vi "Display Options Window.vi"(8 "error in (no error)":errorcluster, 11 "Feed Module State Cluster in":T1={"Shared Variables"={"PID 1 Process Variable"="PID1-Mettler Toledo Scale 1", "PID 1 Output"="PID1-Mettler Toledo Scale 1", "PID 1 Setpoint"="PID1-Setpoint", "PID 1 Setpoint SV refnum"="ni.var.psp://localhost/Flow Module 1/PID1-Setpoint", "PID 1 Process Variable SV refnum"="ni.var.psp://localhost/Flow Module 1/PID1-Setpoint", "PID 1 Output SV refnum"="ni.var.psp://localhost/Flow Module 1/PID1-Setpoint"}, "Feed Module Config"={"GUID"="", "Drop Coords"={"Horizontal"=0, "Vertical"=0}, "Process Name"="", "User name"="", "Queue Name"="", "Settings"={"Cycle Period"=500.0, "Ismatech"={"VISA resource name"="", "Simulated?"=TRUE, "Pump Number"=1.0, "Reverse?"=FALSE}, "Masterflex"={"VISA resource name"="", "Simulated?"=TRUE, "Pump Number"=1.0, "Reverse?"=FALSE}, "Mettler"={"VISA resource name"="", "Simulated?"=FALSE}, "Bronkhorst M13 Flow Meter"={"VISA resource name"="", "Simulated?"=TRUE, "Smoothing Steps"=1}, "PID 2 Parameters"={"Input Device"=enum."Default", "Output Device"=enum."Default", "Setpoint"=0.0, "PID gains"={"proportional gain (Kc)"=1.0, "integral time (Ti, min)"=0.01, "derivative time (Td, min)"=0.0}}, "Manual Entry"=0.0, "Auto?"=TRUE, "PID range"={"PID High"=100.0, "PID Low"=0.0, "High Warning"=100.0}, "Tacmina Settings"={"Analog DAQ Task"="", "Digital DAQ Task"=""}, "KNF SIMDOS Settings"={"VISA resource name"="", "Simulated?"=TRUE}, "ASIA Pump C"={"ASIA Pump #"=0, "channel"=0, "Simulated"=FALSE}, "VICI Settings"={"VISA resource name"="", "Pump ID"="", "Pump Head Vol"=0.0, "Reverse?"=FALSE, "Simulated?"=TRUE}, "FLOM Settings"={"VISA resource name"="", "Simulated?"=TRUE, "Pump Number"=0.0}, "SSI PR/LD Settings"={"VISA resource name"="", "Simulated?"=FALSE}, "Masterflex 75211 Settings"={"Analog DAQ Task"="", "Digital DAQ Task"=""}, "SSI P40 Settings"={"VISA resource name"="", "Simulated?"=TRUE}, "Ismatech 3 Channel Settings"={"VISA resource name"="", "Pump Number"=1, "Channel Number"=0, "Simulated?"=TRUE, "Reverse?"=FALSE}, "Bronkhorst M14 Settings"={"VISA resource name"="", "Simulated?"=FALSE, "Smoothing Steps"=1}, "Reset Totalizer"=FALSE, "Input Num Alarm Settings"=[], "Control Type"=enum."g/min", "Front End Display Options"={"Temperature"=TRUE, "Scale Grams"=FALSE, "Density"=TRUE, "Flow (g/min)"=FALSE, "Flow (ml/min)"=TRUE, "PSIG"=TRUE, "Total Grams"=TRUE, "Updated"=TRUE}}, "Settings Load Count"=0, "OP Load Count"=0}} {"Feed Module Config"."Settings"."Bronkhorst M14 Settings"."Smoothing Steps" min=1 step=1; "Feed Module Config"."Settings"."Ismatech 3 Channel Settings"."Channel Number" min=0 max=3; "Feed Module Config"."Settings"."Ismatech 3 Channel Settings"."Pump Number" min=1; "Feed Module Config"."Settings"."PID range"."PID Low" min=0.0 max=100.0 format="%.2f"; "Feed Module Config"."Settings"."PID range"."PID High" format="%.2f"; "Feed Module Config"."Settings"."PID 2 Parameters"."PID gains"."derivative time (Td, min)" format="%.3f"; "Feed Module Config"."Settings"."PID 2 Parameters"."PID gains"."integral time (Ti, min)" format="%.3f"; "Feed Module Config"."Settings"."PID 2 Parameters"."PID gains"."proportional gain (Kc)" format="%.3f"; "Feed Module Config"."Settings"."Bronkhorst M13 Flow Meter"."Smoothing Steps" min=1 step=1; "Feed Module Config"."Settings"."ASIA Pump C"."channel" min=0 max=1 step=1; "Feed Module Config"."Settings"."Ismatech"."Pump Number" min=1.0 max=20.0 step=1.0; "Feed Module Config"."Settings"."Masterflex"."Pump Number" min=1.0 max=20.0 step=1.0}) -> (0 "error out":errorcluster, 2 "Updated in DO":bool, 3 "Feed Module State Cluster out":T1={"Shared Variables"={"PID 1 Process Variable"="PID1-Mettler Toledo Scale 1", "PID 1 Output"="PID1-Mettler Toledo Scale 1", "PID 1 Setpoint"="PID1-Setpoint", "PID 1 Setpoint SV refnum"="ni.var.psp://localhost/Flow Module 1/PID1-Setpoint", "PID 1 Process Variable SV refnum"="ni.var.psp://localhost/Flow Module 1/PID1-Setpoint", "PID 1 Output SV refnum"="ni.var.psp://localhost/Flow Module 1/PID1-Setpoint"}, "Feed Module Config"={"GUID"="", "Drop Coords"={"Horizontal"=0, "Vertical"=0}, "Process Name"="", "User name"="", "Queue Name"="", "Settings"={"Cycle Period"=500.0, "Ismatech"={"VISA resource name"="", "Simulated?"=TRUE, "Pump Number"=1.0, "Reverse?"=FALSE}, "Masterflex"={"VISA resource name"="", "Simulated?"=TRUE, "Pump Number"=1.0, "Reverse?"=FALSE}, "Mettler"={"VISA resource name"="", "Simulated?"=FALSE}, "Bronkhorst M13 Flow Meter"={"VISA resource name"="", "Simulated?"=TRUE, "Smoothing Steps"=1}, "PID 2 Parameters"={"Input Device"=enum."Default", "Output Device"=enum."Default", "Setpoint"=0.0, "PID gains"={"proportional gain (Kc)"=1.0, "integral time (Ti, min)"=0.01, "derivative time (Td, min)"=0.0}}, "Manual Entry"=0.0, "Auto?"=TRUE, "PID range"={"PID High"=100.0, "PID Low"=0.0, "High Warning"=100.0}, "Tacmina Settings"={"Analog DAQ Task"="", "Digital DAQ Task"=""}, "KNF SIMDOS Settings"={"VISA resource name"="", "Simulated?"=TRUE}, "ASIA Pump C"={"ASIA Pump #"=0, "channel"=0, "Simulated"=FALSE}, "VICI Settings"={"VISA resource name"="", "Pump ID"="", "Pump Head Vol"=0.0, "Reverse?"=FALSE, "Simulated?"=TRUE}, "FLOM Settings"={"VISA resource name"="", "Simulated?"=TRUE, "Pump Number"=0.0}, "SSI PR/LD Settings"={"VISA resource name"="", "Simulated?"=FALSE}, "Masterflex 75211 Settings"={"Analog DAQ Task"="", "Digital DAQ Task"=""}, "SSI P40 Settings"={"VISA resource name"="", "Simulated?"=TRUE}, "Ismatech 3 Channel Settings"={"VISA resource name"="", "Pump Number"=1, "Channel Number"=0, "Simulated?"=TRUE, "Reverse?"=FALSE}, "Bronkhorst M14 Settings"={"VISA resource name"="", "Simulated?"=FALSE, "Smoothing Steps"=1}, "Reset Totalizer"=FALSE, "Input Num Alarm Settings"=[], "Control Type"=enum."g/min", "Front End Display Options"={"Temperature"=TRUE, "Scale Grams"=FALSE, "Density"=TRUE, "Flow (g/min)"=FALSE, "Flow (ml/min)"=TRUE, "PSIG"=TRUE, "Total Grams"=TRUE, "Updated"=TRUE}}, "Settings Load Count"=0, "OP Load Count"=0}} {"Feed Module Config"."Settings"."Bronkhorst M14 Settings"."Smoothing Steps" min=1 step=1; "Feed Module Config"."Settings"."Ismatech 3 Channel Settings"."Channel Number" min=0 max=3; "Feed Module Config"."Settings"."Ismatech 3 Channel Settings"."Pump Number" min=1; "Feed Module Config"."Settings"."PID range"."PID Low" min=0.0 max=100.0 format="%.2f"; "Feed Module Config"."Settings"."PID range"."PID High" format="%.2f"; "Feed Module Config"."Settings"."PID 2 Parameters"."PID gains"."derivative time (Td, min)" format="%.3f"; "Feed Module Config"."Settings"."PID 2 Parameters"."PID gains"."integral time (Ti, min)" format="%.3f"; "Feed Module Config"."Settings"."PID 2 Parameters"."PID gains"."proportional gain (Kc)" format="%.3f"; "Feed Module Config"."Settings"."Bronkhorst M13 Flow Meter"."Smoothing Steps" min=1 step=1; "Feed Module Config"."Settings"."ASIA Pump C"."channel" min=0 max=1 step=1; "Feed Module Config"."Settings"."Ismatech"."Pump Number" min=1.0 max=20.0 step=1.0; "Feed Module Config"."Settings"."Masterflex"."Pump Number" min=1.0 max=20.0 step=1.0})   [LabVIEW 2018, in "Feed Module.lvlib"]
uses:
  Feed Module.lvlib
  Controls/Feed Module Front End Display Options.ctl
  Controls/Feed Module State Cluster.ctl
  Controls/Feed Module Shared Variable Cluster.ctl
  Controls/Feed Module Config Cluster.ctl
  <vilib>/Utility/miscctls.llb/LVPoint32TypeDef.ctl
  Controls/Feed Module Settings Cluster.ctl
  Ismatec ISM 831C/Controls/Ismatech ISM831C Settings Cluster.ctl
  Masterflex 7550-30/Controls/Settings Cluster.ctl
  Mettler Toledo/Controls/Settings Cluster.ctl
  Bronkhorst M13 Flow Meter/Settings Cluster.ctl
  Measure Instrument/PID 2 Parameters Cluster.ctl
  Measure Instrument/PID Input Enum.ctl
  Measure Instrument/PID 2 Output Enum.ctl
  Tacmina QI/Tacmina QI DAQ Setting.ctl
  KNF Pump/Settings Cluster plus SIMDOS.ctl
  ASIA Pump/Pump Settings.ctl
  VICI M50 Party Mode/Settings Cluster.ctl
  FLOM Pump/Settings Cluster.ctl
  SSI PR Class/SSI PR or LD Settings Cluster.ctl
  Masterflex 75211/Masterflex 75211 DAQ Setting.ctl
  SSI PR Class/SSI P40 Settings Cluster.ctl
  Ismatec 78001/Ismatec 4083.ctl
  Bronkhorst M14 Flow Meter/Settings Cluster.ctl
  Tag VIs/Numeric Alarm Settings Cluster.ctl
  Masterflex 75211/Masterflex 75211.lvlib
  Masterflex 7550-30/Masterflex 7550-30.lvlib
  Ismatec ISM 831C/Ismatec ISM 831C.lvlib
  Tacmina QI/Tacmina QI.lvlib
  KNF Pump/KNF SIMDOS.lvlib
  VICI M50 Party Mode/VICI M6 M50 Party Mode.lvlib
  FLOM Pump/FLOM Pump.lvlib
  ASIA Pump.lvlib
  Mettler Toledo/Mettler Toledo.lvlib
  Bronkhorst M13 Flow Meter/Bronkhorst M13 Flow Meter.lvlib
  SSI PR Class/SSI PR or LD Pump.lvlib
  SSI PR Class/SSI P40 Pump.lvlib
  Ismatec 78001/Ismatec 4308.lvlib
  Bronkhorst M14 Flow Meter/Bronkhorst M14 Flow Meter.lvlib
panel:
  in  "Cancel Button":bool
  in  "OK Button":bool
  in  "Front End Display Options":T24
  # "Output Instruments"
  # "Input Instruments"
  # "Output Instruments"
  # "Input Instruments"
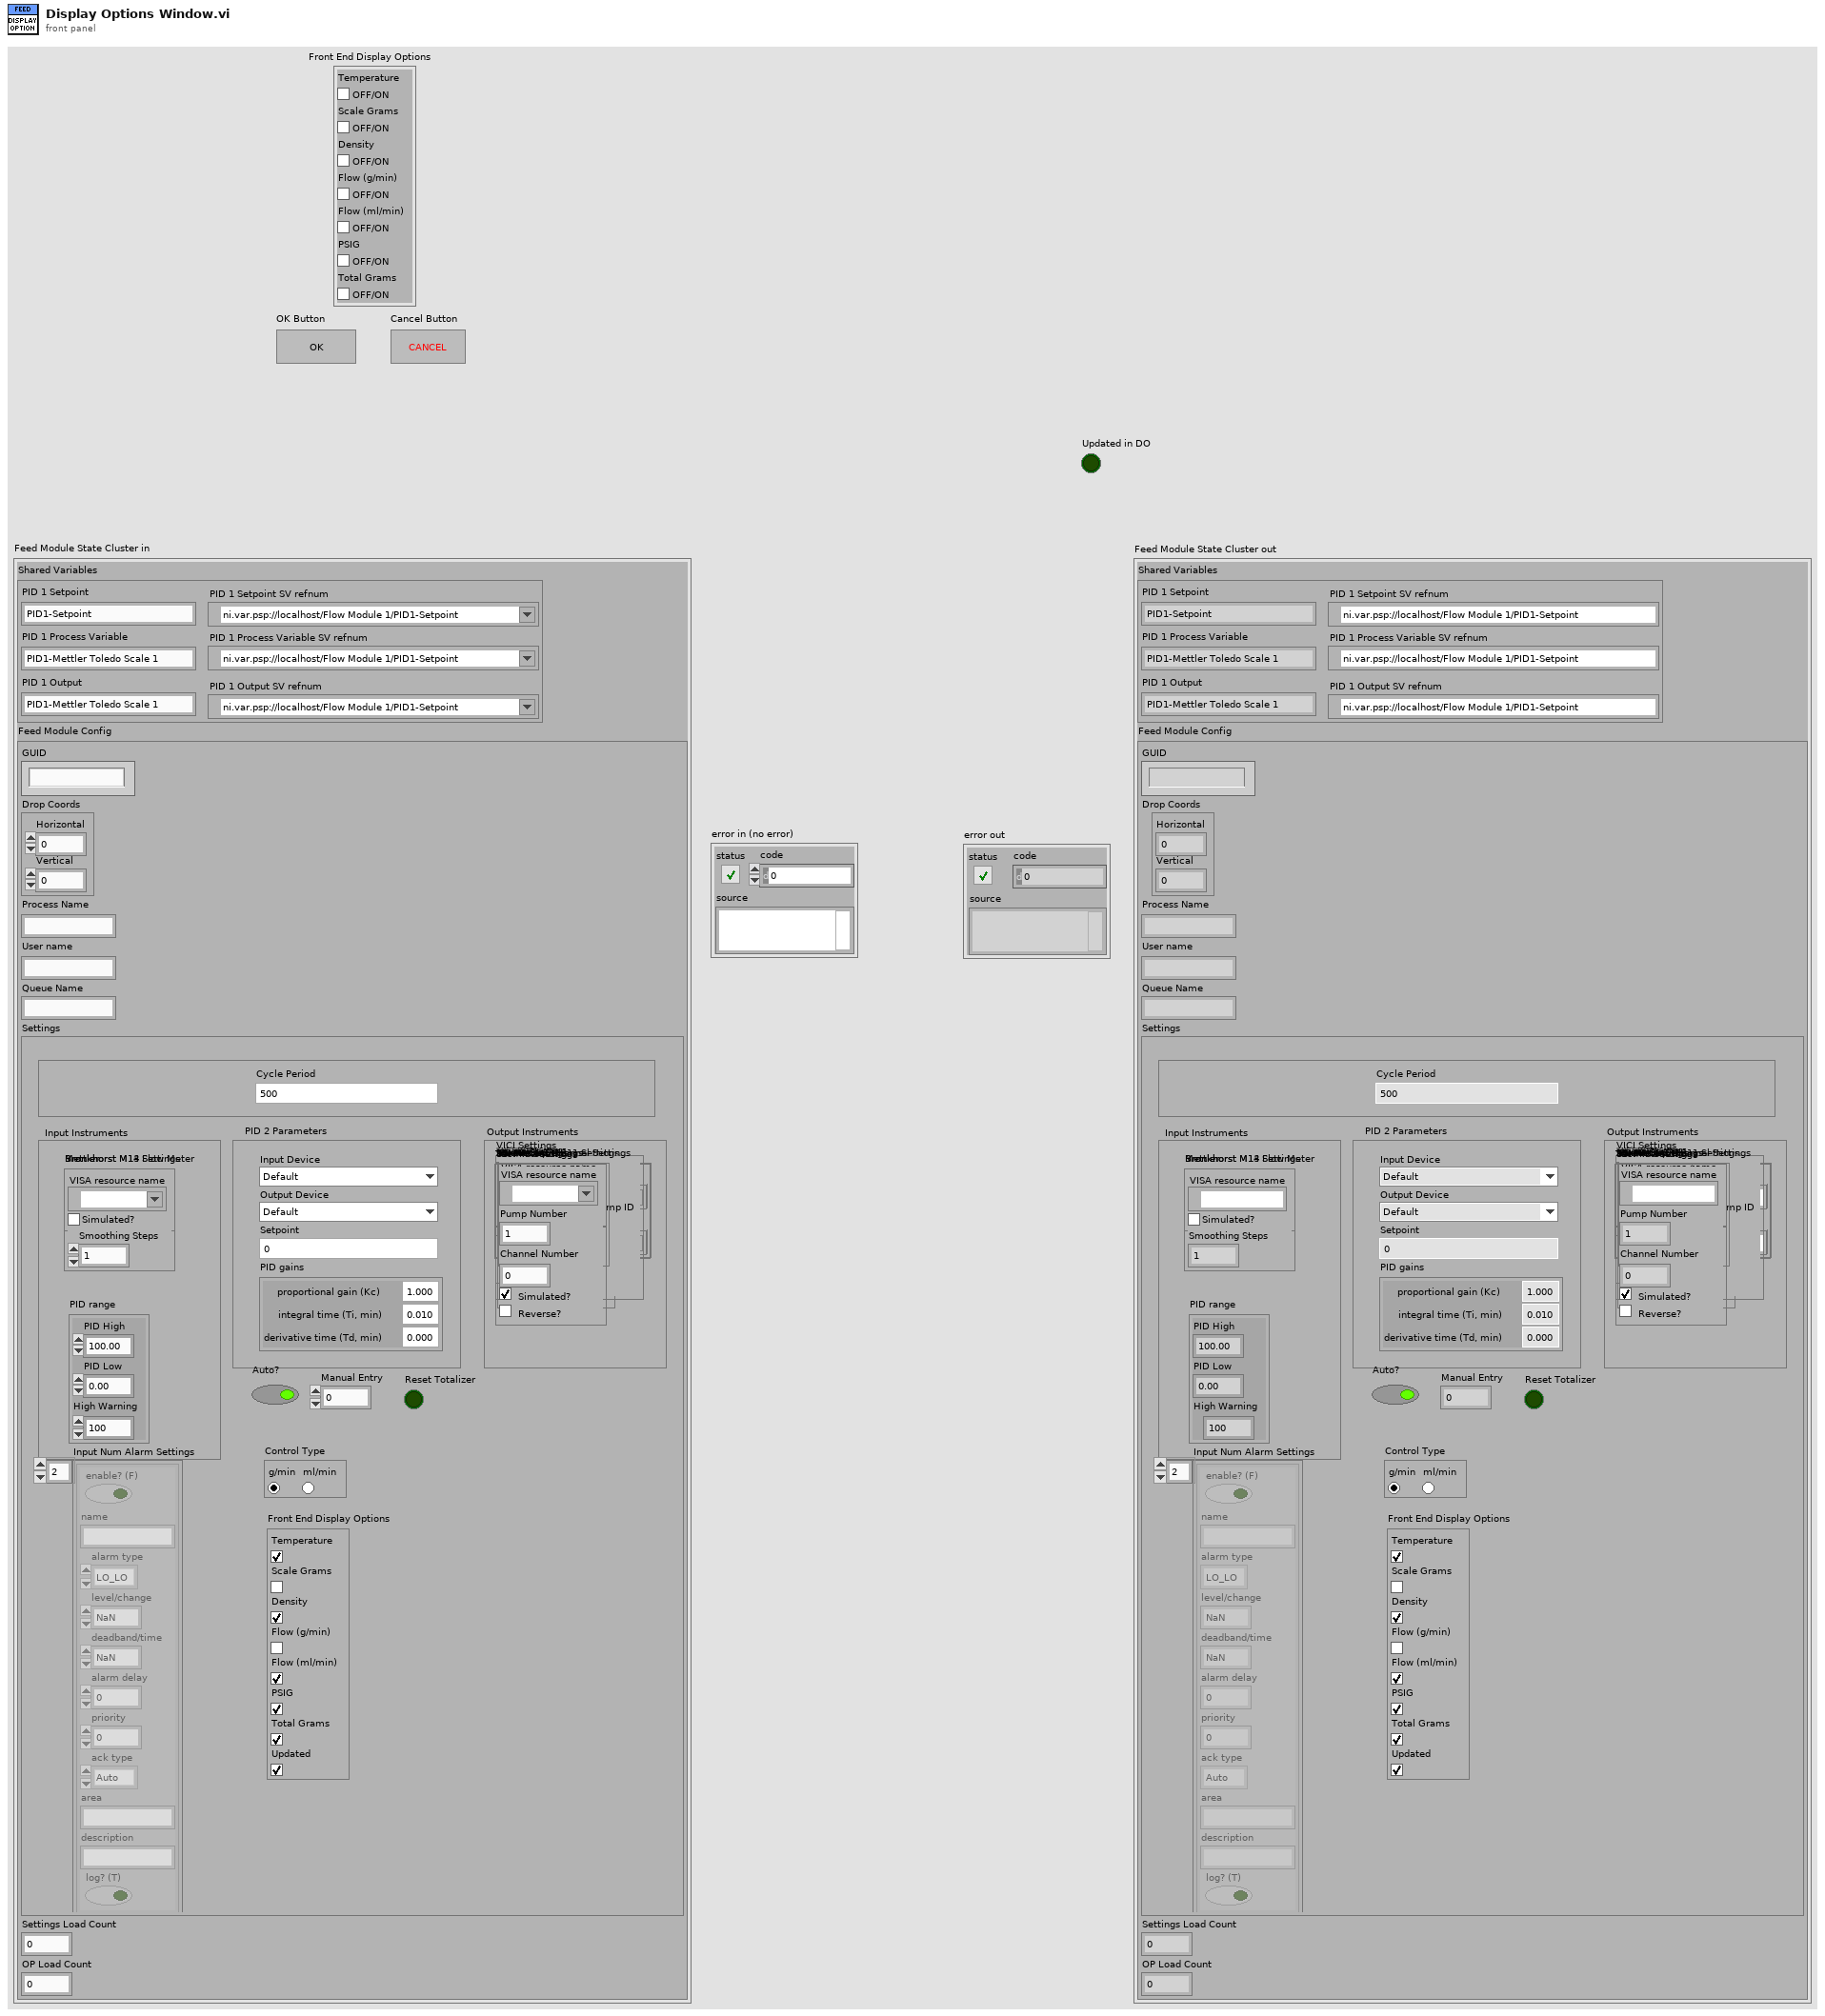
[diagram p1: front panel]
types:
  T1 = typedef "Feed Module.lvlib/Feed Module State Cluster.ctl" = cluster{"Shared Variables":T2, "Feed Module Config":T3}
  T2 = typedef "Feed Module.lvlib/Feed Module Shared Variable Cluster.ctl" = cluster{"PID 1 Process Variable":string, "PID 1 Output":string, "PID 1 Setpoint":string, "PID 1 Setpoint SV refnum":refnum<k21>, "PID 1 Process Variable SV refnum":refnum<k21>, "PID 1 Output SV refnum":refnum<k21>}
  T3 = typedef "Feed Module.lvlib/Feed Module Config Cluster.ctl" = cluster{"GUID":string, "Drop Coords":T4, "Process Name":string, "User name":string, "Queue Name":string, "Settings":T5, "Settings Load Count":i32, "OP Load Count":i32}
  T4 = typedef "LVPoint32TypeDef.ctl" = cluster{"Horizontal":i32, "Vertical":i32}
  T5 = typedef "Feed Module.lvlib/Feed Module Settings Cluster.ctl" = cluster{"Cycle Period":dbl, "Ismatech":T6, "Masterflex":T7, "Mettler":T8, "Bronkhorst M13 Flow Meter":T9, "PID 2 Parameters":T10, "Manual Entry":dbl, "Auto?":bool, "PID range":cluster{"PID High":dbl, "PID Low":dbl, "High Warning":dbl}, "Tacmina Settings":T13, "KNF SIMDOS Settings":T14, "ASIA Pump C":T15, "VICI Settings":T16, "FLOM Settings":T17, "SSI PR/LD Settings":T18, "Masterflex 75211 Settings":T19, "SSI P40 Settings":T20, "Ismatech 3 Channel Settings":T21, "Bronkhorst M14 Settings":T22, "Reset Totalizer":bool, "Input Num Alarm Settings":T23[], "Control Type":enum32{"g/min", "ml/min"}, "Front End Display Options":cluster{"Temperature":bool, "Scale Grams":bool, "Density":bool, "Flow (g/min)":bool, "Flow (ml/min)":bool, "PSIG":bool, "Total Grams":bool, "Updated":bool}}
  T6 = typedef "Ismatec ISM 831C.lvlib/Ismatech ISM831C Settings Cluster.ctl" = cluster{"VISA resource name":refnum<visa-resource-name>, "Simulated?":bool, "Pump Number":dbl, "Reverse?":bool}
  T7 = typedef "Masterflex 7550-30.lvlib/Settings Cluster.ctl" = cluster{"VISA resource name":refnum<visa-resource-name>, "Simulated?":bool, "Pump Number":dbl, "Reverse?":bool}
  T8 = typedef "Mettler Toledo.lvlib/Settings Cluster.ctl" = cluster{"VISA resource name":refnum<visa-resource-name>, "Simulated?":bool}
  T9 = typedef "Bronkhorst M13 Flow Meter.lvlib/Settings Cluster.ctl" = cluster{"VISA resource name":refnum<visa-resource-name>, "Simulated?":bool, "Smoothing Steps":i32}
  T10 = typedef "PID 2 Parameters Cluster.ctl" = cluster{"Input Device":T11, "Output Device":T12, "Setpoint":dbl, "PID gains":cluster{"proportional gain (Kc)":dbl, "integral time (Ti, min)":dbl, "derivative time (Td, min)":dbl}}
  T11 = typedef "PID Input Enum.ctl" = enum16{"Default", "Bronkhorst M13", "Bronkhorst M14", "Scale Rate of Change"}
  T12 = typedef "PID 2 Output Enum.ctl" = enum16{"Default", "Ismatec ISM 4308", "Ismatec ISM 831C", "Masterflex 7550-30", "VICI M6", "VICI M50", "Tacmina QI", "KNF SIMDOS", "ASIA Type C", "FLOM UI-22-11", "SSI PR/LD", "SSI P40", "Masterflex 75211-70"}
  T13 = typedef "Tacmina QI.lvlib/Tacmina QI DAQ Setting.ctl" = cluster{"Analog DAQ Task":refnum<k21>, "Digital DAQ Task":refnum<k21>}
  T14 = typedef "KNF SIMDOS.lvlib/Settings Cluster plus SIMDOS.ctl" = cluster{"VISA resource name":refnum<visa-resource-name>, "Simulated?":bool}
  T15 = typedef "ASIA Pump.lvlib/Pump Settings.ctl" = cluster{"ASIA Pump #":i32, "channel":i32, "Simulated":bool}
  T16 = typedef "VICI M6 M50 Party Mode.lvlib/Settings Cluster.ctl" = cluster{"VISA resource name":refnum<visa-resource-name>, "Pump ID":string, "Pump Head Vol":dbl, "Reverse?":bool, "Simulated?":bool}
  T17 = typedef "FLOM Pump.lvlib/Settings Cluster.ctl" = cluster{"VISA resource name":refnum<visa-resource-name>, "Simulated?":bool, "Pump Number":dbl}
  T18 = typedef "SSI PR or LD Pump.lvlib/SSI PR or LD Settings Cluster.ctl" = cluster{"VISA resource name":refnum<visa-resource-name>, "Simulated?":bool}
  T19 = typedef "Masterflex 75211.lvlib/Masterflex 75211 DAQ Setting.ctl" = cluster{"Analog DAQ Task":refnum<k21>, "Digital DAQ Task":refnum<k21>}
  T20 = typedef "SSI P40 Pump.lvlib/SSI P40 Settings Cluster.ctl" = cluster{"VISA resource name":refnum<visa-resource-name>, "Simulated?":bool}
  T21 = typedef "Ismatec 4308.lvlib/Ismatec 4083.ctl" = cluster{"VISA resource name":refnum<visa-resource-name>, "Pump Number":i16, "Channel Number":i16, "Simulated?":bool, "Reverse?":bool}
  T22 = typedef "Bronkhorst M14 Flow Meter.lvlib/Settings Cluster.ctl" = cluster{"VISA resource name":refnum<visa-resource-name>, "Simulated?":bool, "Smoothing Steps":i32}
  T23 = typedef "Numeric Alarm Settings Cluster.ctl" = cluster{"enable? (F)":bool, "name":string, "alarm type":enum16{"HI_HI", "HI", "LO", "LO_LO"}, "level/change":dbl, "deadband/time":dbl, "alarm delay":dbl, "priority":u32, "ack type":enum16{"Auto", "User", "None", "Each Occurrence"}, "area":string, "description":string, "log? (T)":bool}
  T24 = typedef "Feed Module Front End Display Options.ctl" = cluster{"Temperature":bool, "Scale Grams":bool, "Density":bool, "Flow (g/min)":bool, "Flow (ml/min)":bool, "PSIG":bool, "Total Grams":bool}
  T25 = cluster{"Temperature":bool, "Scale Grams":bool, "Density":bool, "Flow (g/min)":bool, "Flow (ml/min)":bool, "PSIG":bool, "Total Grams":bool, "Updated":bool}
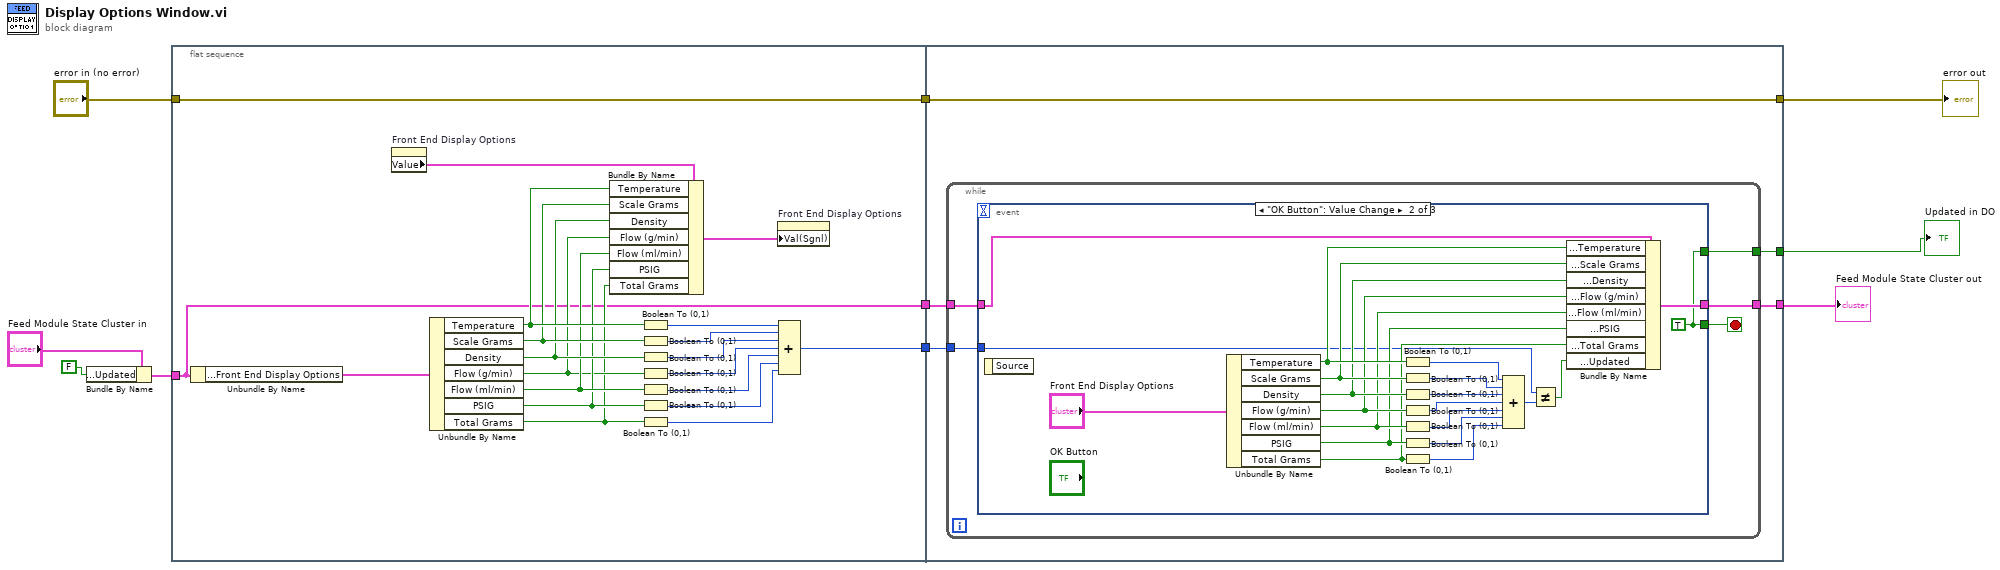
[diagram p0: block diagram]
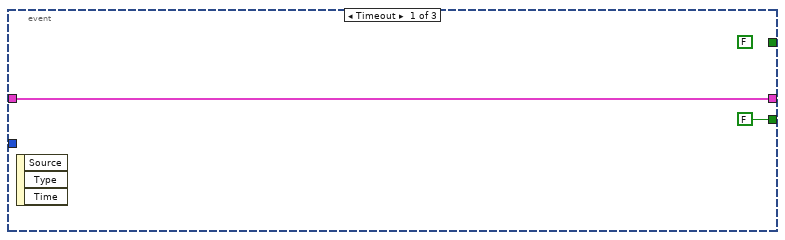
[diagram p2: hidden frame]
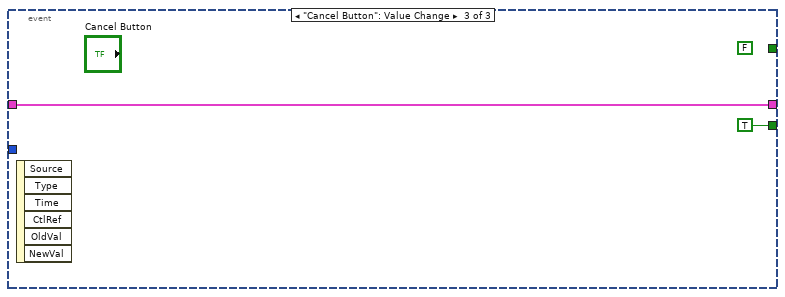
[diagram p3: hidden frame]
diagram:
  n1 = Bundle By Name(cluster="Feed Module State Cluster in", "Feed Module Config.Settings.Front End Display Options.Updated"=FALSE) -> (w5:T1)
  n2 = flat-sequence {
    tunnel: w5 -> [w12]
    tunnel: [w12] -> w9
    tunnel: [w15] -> w4
    tunnel: "error in (no error)" -> [w11]
    tunnel: [w11] -> w2
    tunnel: [w32] -> w10
    tunnel: w9 -> [w35]
    tunnel: [w34] -> w8
    tunnel: w4 -> [w33]
    tunnel: w2 -> [w32]
    tunnel: [w31] -> w1
    frame #0 {
      n3 = Unbundle By Name(w12) -> ("Feed Module Config.Settings.Front End Display Options"=w30:T25)
      n4 = property on="Front End Display Options" class="Clust (strict)"() -> ("Value"=w13:T24)  [unwired: 2 in, 2 out]
      n5 = Unbundle By Name(w30) -> ("Temperature"=w23:bool, "Scale Grams"=w22:bool, "Density"=w21:bool, "Flow (g/min)"=w18:bool, "Flow (ml/min)"=w20:bool, "PSIG"=w19:bool, "Total Grams"=w16:bool)
      n6 = Bundle By Name(cluster=w13, "Temperature"=w23, "Scale Grams"=w22, "Density"=w21, "Flow (g/min)"=w18, "Flow (ml/min)"=w20, "PSIG"=w19, "Total Grams"=w16) -> (w14:T24)
      n7 = Boolean To (0,1)(Boolean=w23) -> (0, 1=w29:i16)
      n8 = Boolean To (0,1)(Boolean=w22) -> (0, 1=w28:i16)
      n9 = Boolean To (0,1)(Boolean=w21) -> (0, 1=w27:i16)
      n10 = Boolean To (0,1)(Boolean=w18) -> (0, 1=w26:i16)
      n11 = Boolean To (0,1)(Boolean=w20) -> (0, 1=w25:i16)
      n12 = Boolean To (0,1)(Boolean=w19) -> (0, 1=w24:i16)
      n13 = Boolean To (0,1)(Boolean=w16) -> (0, 1=w17:i16)
      n14 = property on="Front End Display Options" class="Clust (strict)"("Val(Sgnl)"=w14) -> ()  [unwired: 2 in, 2 out]
      n15 = Compound Arithmetic op=ADD(w29, w28, w27, w26, w25, w24, w17) -> (w15:i16)
    }
    frame #1 {
      n16 = while {
        tunnel: w35 -> [w39]
        tunnel: [w38] -> w34
        tunnel: w33 -> [w37]
        tunnel: [w36] -> w31
        stop <- w40 stop-if-true
        n17 = event shown="[1] \"OK Button\": Value Change" {
          selector: _ -> [_ _ _]
          dyn-events: _ -> [_ _ _]
          timeout: _ -> [_ _ _]
          tunnel: [FALSE ("Cancel Button") w43 TRUE ("Cancel Button")] -> w40
          tunnel: w39 -> [w41 w62 w64]
          tunnel: [w41 w61 w64] -> w38
          tunnel: w37 -> [_ w46 _]
          tunnel: [_ w43 _] -> w36
          event Timeout {
            (unwired) FALSE
            n18 = event-data() -> ()  [unwired: 1 in, 3 out]
          }
          event "OK Button": Value Change {
            w43 = TRUE ("Cancel Button")
            n19 = event-data() -> ()  [unwired: 1 in, 1 out]
            n20 = Unbundle By Name("Front End Display Options") -> ("Temperature"=w53:bool, "Scale Grams"=w52:bool, "Density"=w51:bool, "Flow (g/min)"=w50:bool, "Flow (ml/min)"=w49:bool, "PSIG"=w48:bool, "Total Grams"=w47:bool)
            n21 = Boolean To (0,1)(Boolean=w53) -> (0, 1=w60:i16)
            n22 = Boolean To (0,1)(Boolean=w52) -> (0, 1=w59:i16)
            n23 = Boolean To (0,1)(Boolean=w51) -> (0, 1=w58:i16)
            n24 = Boolean To (0,1)(Boolean=w50) -> (0, 1=w57:i16)
            n25 = Boolean To (0,1)(Boolean=w49) -> (0, 1=w56:i16)
            n26 = Boolean To (0,1)(Boolean=w48) -> (0, 1=w55:i16)
            n27 = Boolean To (0,1)(Boolean=w47) -> (0, 1=w54:i16)
            n28 = Compound Arithmetic op=ADD(w60, w59, w58, w57, w56, w55, w54) -> (w45:i16)
            n29 = Not Equal?(x=w46, y=w45) -> (x != y?=w44:bool)
            n30 = Bundle By Name(cluster=w62, "Feed Module Config.Settings.Front End Display Options.Temperature"=w53, "Feed Module Config.Settings.Front End Display Options.Scale Grams"=w52, "Feed Module Config.Settings.Front End Display Options.Density"=w51, "Feed Module Config.Settings.Front End Display Options.Flow (g/min)"=w50, "Feed Module Config.Settings.Front End Display Options.Flow (ml/min)"=w49, "Feed Module Config.Settings.Front End Display Options.PSIG"=w48, "Feed Module Config.Settings.Front End Display Options.Total Grams"=w47, "Feed Module Config.Settings.Front End Display Options.Updated"=w44) -> (w61:T1)
          }
          event "Cancel Button": Value Change {
            (unwired) FALSE
            n31 = event-data() -> ()  [unwired: 1 in, 6 out]
          }
        }
      }
    }
  }
  "error out" <- w10
  "Feed Module State Cluster out" <- w8
  "Updated in DO" <- w1
